vi "MakeSnakeTailLonger.vi"(0 "object in":refnum<class "Game Board.lvclass">, 5 "error in (no error)":errorcluster) -> (14 "object out":refnum<class "Game Board.lvclass">, 19 "error out":errorcluster)   [LabVIEW 2021, in "Game Board.lvclass"]
uses:
  Game Board.lvclass
  Game Board.lvclass/Game Board.ctl
  Snake_class/Snake.lvclass
  Fruit_class/Fruit.lvclass
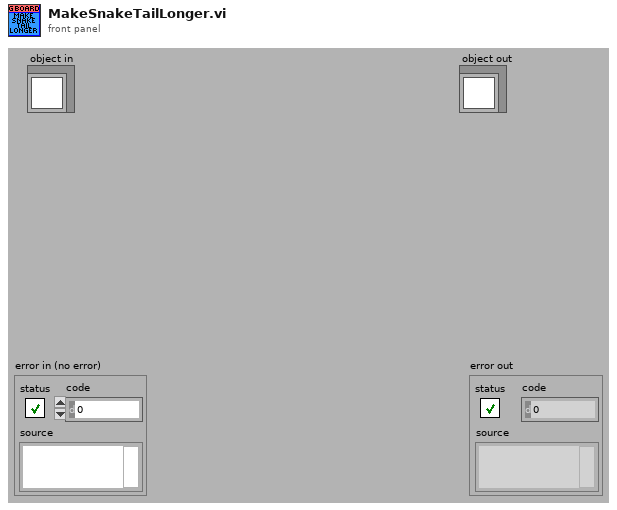
[diagram p1: front panel]
types:
  T1 = typedef "Coordinates.ctl" = cluster{"X":i32, "Y":i32}
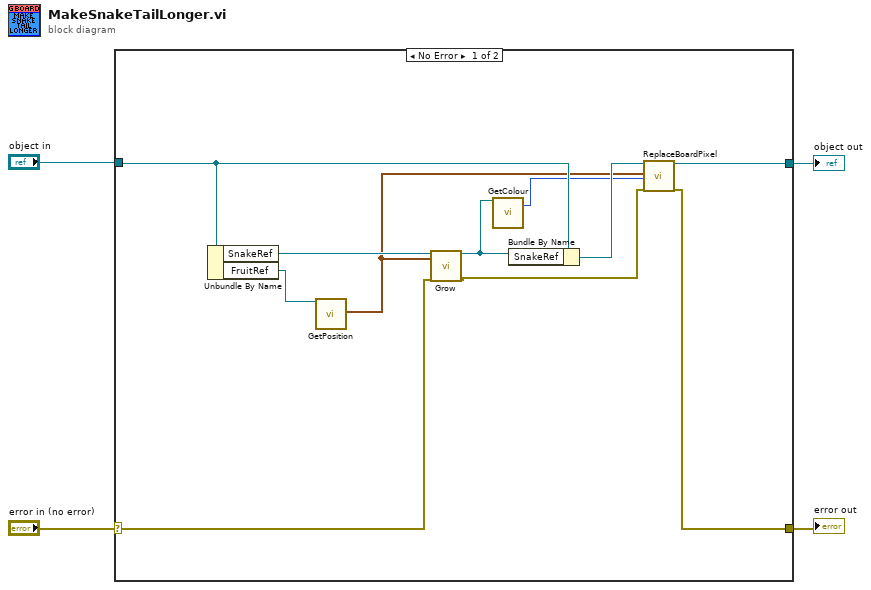
[diagram p0: block diagram]
diagram:
  n1 = case shown="No Error" "error in (no error)" {
    selector: "error in (no error)" -> [w7 w17]
    tunnel: [w5 w17] -> w3
    tunnel: [w12 w16] -> w1
    tunnel: "object in" -> [w15 w16]
    frame No Error {
      n2 = Unbundle By Name(w15) -> ("SnakeRef"=w11:refnum<class "Snake.lvclass">, "FruitRef"=w14:refnum<class "Fruit.lvclass">)
      n3 = call "GetPosition.vi"("object in"=w14) -> ("Coordinates"=w10:T1)  [unwired: 17 in, 1 out]
      n4 = call-dynamic "Grow.vi"("object in"=w11, "Coordinates"=w10, "error in (no error)"=w7) -> ("object out"=w9:refnum<class "Snake.lvclass">, "error out"=w6:errorcluster)  [unwired: 15 in]
      n5 = call-dynamic "GetColour.vi"("object in"=w9) -> ("Colour"=w8:u32)  [unwired: 16 in, 2 out]
      n6 = Bundle By Name(cluster=w15, "SnakeRef"=w9) -> (w13:refnum<class "Game Board.lvclass">)
      n7 = call-dynamic "ReplaceBoardPixel.vi"("object in"=w13, "Coordinates"=w10, "Colour"=w8, "error in (no error)"=w6) -> ("object out"=w12:refnum<class "Game Board.lvclass">, "error out"=w5:errorcluster)  [unwired: 14 in]
    }
    frame Error {
    }
  }
  "error out" <- w3
  "object out" <- w1
